vi "GW AFG2000 Basic Example.vi"() -> ()   [LabVIEW 2017]
panel:
  in  "Frequency (1000 Hz)":dbl=1000.0 min=0.1 max=5000000.0 step=0.1
  out "error out":errorcluster
  in  "DC Offset (0.00 V)":dbl
  in  "UNIT (0:VPP)":u16(ring) items=["Vpp", "Vrms", "dBm"]
  in  "Amplitude (1.0)":dbl=1.0 format="%.1f"
  in  "Waveform Function (0: Sine)":u16(ring) items=["Sine", "Square", "Ramp", "Noise", "USER"]
  in  "VISA resource name":refnum<visa-resource-name>="COM15"
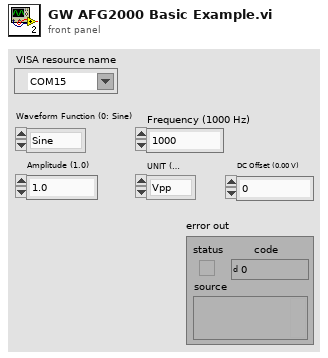
[diagram p1: front panel]
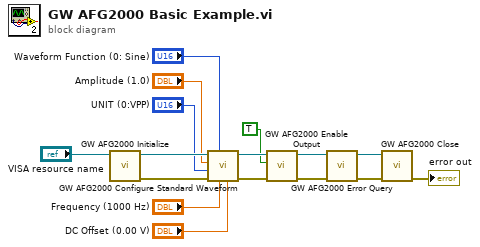
[diagram p0: block diagram]
diagram:
  n1 = call <instrlib>:"GW AFG2000 Initialize.vi"("VISA resource name"="VISA resource name") -> ("error out"=w12:errorcluster, "VISA resource name out"=w13:refnum<visa-resource-name>)  [unwired: 9 in]
  n2 = call <instrlib>:"GW AFG2000 Configure Standard Waveform.vi"("DC Offset (0.00 V)"="DC Offset (0.00 V)", "Frequency (1000 Hz)"="Frequency (1000 Hz)", "Waveform Function (0: Sine)"="Waveform Function (0: Sine)", "error in (no error)"=w12, "UNIT (0:VPP)"="UNIT (0:VPP)", "Amplitude (1.0)"="Amplitude (1.0)", "VISA resource name"=w13) -> ("error out"=w16:errorcluster, "VISA resource name out"=w15:refnum<visa-resource-name>)  [unwired: 3 in]
  n3 = call <instrlib>:"GW AFG2000 Enable Output.vi"("error in (no error)"=w16, "Enable Output (T: Enable)"=TRUE, "VISA resource name"=w15) -> ("error out"=w5:errorcluster, "VISA resource name out"=w6:refnum<visa-resource-name>)  [unwired: 7 in]
  n4 = call <instrlib>:"GW AFG2000 Error Query.vi"("error in (no error)"=w5, "VISA resource name"=w6) -> ("error out"=w3:errorcluster, "VISA resource name out"=w4:refnum<visa-resource-name>)  [unwired: 6 in, 2 out]
  n5 = call <instrlib>:"GW AFG2000 Close.vi"("error in (no error)"=w3, "VISA session"=w4) -> ("error out"=→"error out":errorcluster)  [unwired: 9 in]
